vi "SPC_get_buffer_from_stream.vi"(6 "Stream Handle":i16, 7 "Buffer Size":u32, 8 "Error In":errorcluster, 9 "Free Buffer":i16, 10 "Buffer No":u16, 11 "DLL Path":path) -> (0 "Error Out":errorcluster, 2 "Buffer Size":u32, 3 "DLL Path":path, 4 "Stream Handle":i16, 5 "Data Buffer":u8[](array[numeric]))   [LabVIEW 2023]
doc: "The procedure is used to get contents of stream's internal buffers with photons data to the buffer 'data_buf'. Stream is defined by handle 'stream_hndl'. \nThe procedure works only with 'buffered' streams.\nThe procedure fills 'data_buf' with contents of stream's buffer 'buf_no'.\n'data_buf' must be allocated with minimum 'buf_size' bytes. \nUse SPC_get_stream_buffer_size procedure to get size of buffer 'buf_no', which means the required 'buf_size' value.\nOn exit 'buf_size' is set to real number of bytes copied to 'data_buf'.\nOn demand, the buffer 'buf_no' can be freed on procedure exit, when 'free_buf' parameter equals 1.\nCall SPC_get_phot_stream_info to get info about current number of stream buffers (field no_of_buf of PhotStreamInfo structure). \nBe aware of option FREE_BUF_STREAM ( bit 13 in 'stream_type' parameter while initializing the stream using SPC_init_buf_stream function) It defines a way in which stream's buffers are freed. If it is set, the buffer is freed, when, during SPC_get_photons_from_stream call, all photons from the current buffer are extracted.\nAfter this it will be not possible to get data from it using SPC_get_buffer_from_stream function.\nData taken from stream' buffers can be stored in .spc file for future use ( for example in SPCM application panel 'Convert FIFO files').\nFirst 4 bytes of .spc file it is a header - call SPC_get_fifo_init_vars to get the header value. \nAfter the header, subsequent stream's buffers should be stored.\n\ninfo@becker-hickl.com"
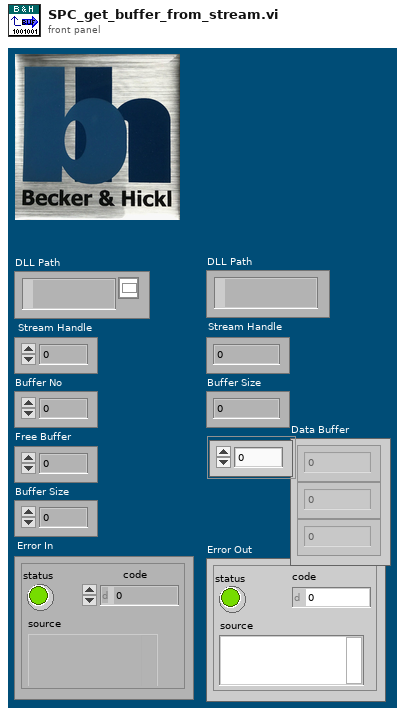
[diagram p1: front panel]
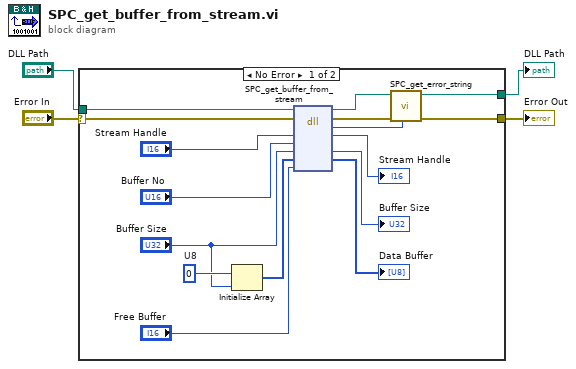
[diagram p0: block diagram]
diagram:
  n1 = case shown="No Error" "Error In" {
    selector: "Error In" -> [w13 w22]
    tunnel: "DLL Path" -> [w16 w21]
    tunnel: [w14 w22] -> w3
    tunnel: [w11 w21] -> w2
    frame No Error {
      w7 = u8 0  # U8
      n2 = Initialize Array(w7, "Buffer Size") -> (w5:u8[])
      n3 = dll-call lib="D:/spcm/lib/lab_view/lv10.0/spcm32.dll" fn="SPC_get_buffer_from_stream"(path in=w16, error in=w13, "stream_hndl"="Stream Handle", "buf_no"="Buffer No", "buf_size"="Buffer Size", "data_buf"=w5, "free_buf"="Free Buffer") -> (path out=w12:path, error out=w15:errorcluster, "return type"=w9:i16, "stream_hndl"=→"Stream Handle":i16, "buf_size"=→"Buffer Size":u32, "data_buf"=→"Data Buffer":u8[])  [unwired: 3 in]
      n4 = call "SPC_get_error_string.vi"("ErrorID"=w9, "Error In"=w15, "DLL Path"=w12) -> ("Error Out"=w14:errorcluster, "DLL Path"=w11:path)  [unwired: 6 in, 1 out]
    }
    frame Error {
    }
  }
  "DLL Path" <- w2
  "Error Out" <- w3
